vi "filter_frequency_imp_test_v10_p.vi"() -> ()   [LabVIEW 2014]
uses:
  <vilib>/rvi/Analysis/host/Butterworth/config/Butterworth Filter Order.ctl
  <vilib>/rvi/Analysis/host/Butterworth/config/Butterworth Filter Type.ctl
  <vilib>/FPGAPlugInAG/cRIO-9039/niLvFpga_Open_cRIO-9039.vi
  <vilib>/rvi/interface/common/dynamic/niFpgaDynamicAddResources.vi
  <vilib>/rvi/Analysis/host/Butterworth/config/BwScaledCoefficients.vi
  <vilib>/Utility/error.llb/Error Cluster From Error Code.vi
  <vilib>/rvi/errors/niLvFpgaAdjustHostInterfaceError.vi
  <vilib>/FPGAPlugInAG/Dynamic/niLvFpga_Close_Dynamic.vi
  <vilib>/rvi/interface/nirviOpenFPGA/nirviOpenFPGA.xnode
  FPGA Bitfiles/test0304_FPGATarget_imptestv10p1_N8vwftCNm6Q.lvbitx
  FPGA VIs/imp_test_v10_p1.vi
  <vilib>/rvi/Analysis/host/Butterworth/XNode/ButterworthCoefficients.xnode
  <vilib>/rvi/interface/nirviReadWriteControl/nirviReadWriteControl.xnode
  <vilib>/rvi/interface/nirviCloseFPGA/nirviCloseFPGA.xnode
  <vilib>/rvi/Analysis/host/Public/NI_FpgaMspHost.lvlib
  NiFpgaLv.dll
  <vilib>/rvi/interface/Simulation/niFpgaSimulationCallBeginRW.vi
panel:
  in  "sr_omega_p_Mavg (S/s)":dbl=50000.0
  in  "fcu_omega_p_Mavg (Hz)":dbl=1000.0
  in  "Filter set":bool
  in  "sr_Strain(Avg.8)_p (S/s)":dbl=50000.0
  in  "fcu_Strain(Avg.8)_p (Hz)":dbl=1000.0
  in  "sr_Dp_dd (S/s)":dbl=50000.0
  in  "fcu_Dp_dd (Hz)":dbl=1000.0
  in  "sr_dFp_PIS (S/s)":dbl=50000.0
  in  "fcu_dFp_PID (Hz)":dbl=1000.0
  in  "sr_Strain(Avg.8)_y (S/s)":dbl=50000.0
  in  "fcu_Strain(Avg.8)_y (Hz)":dbl=1000.0
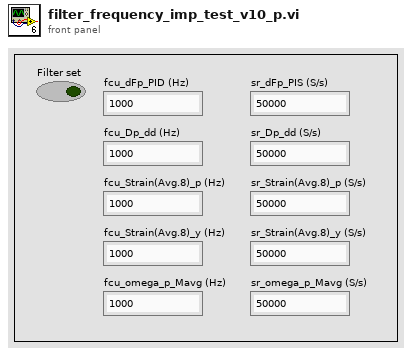
[diagram p1: front panel]
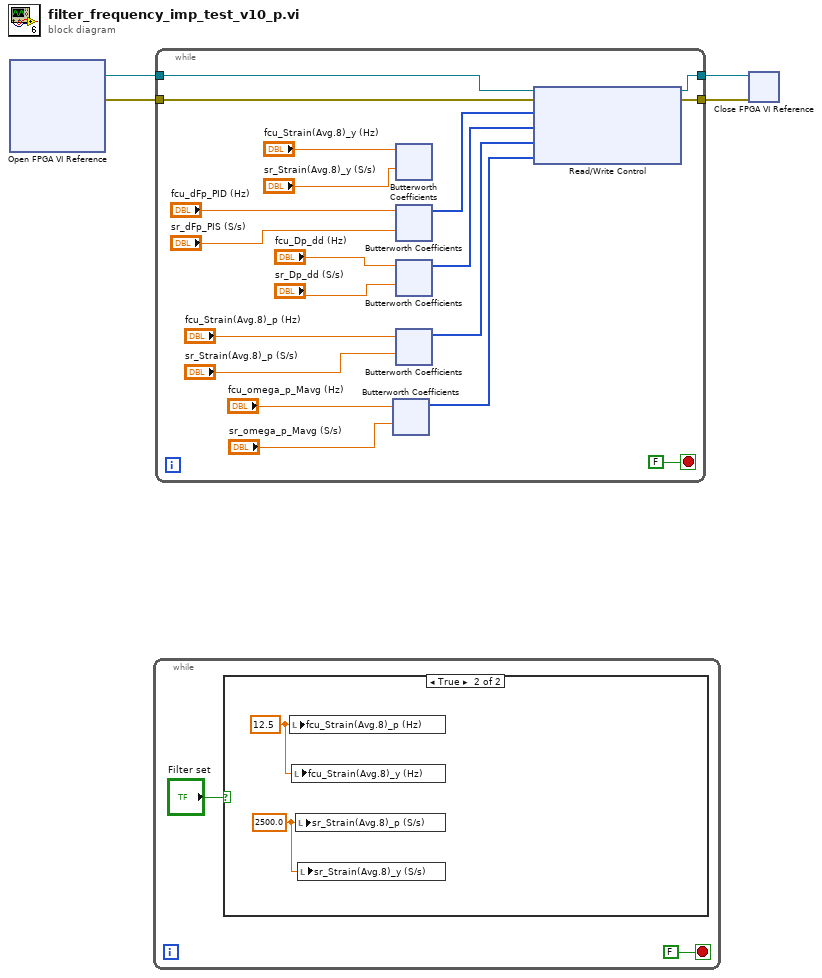
[diagram p0: block diagram]
diagram:
  n1 = xnode "Open FPGA VI Reference"() -> ("FPGA VI Reference Out"=w4:refnum<k20>, "error out"=w3:errorcluster)  [unwired: 2 in]
  n2 = while {
    stop <- FALSE stop-if-true
    n3 = case shown="True" "Filter set" {
      frame False {
      }
      frame True {
        w7 = 2500.0 ("sr_Strain(Avg.8)_p (S/s)")
        w8 = 12.5 ("fcu_Strain(Avg.8)_p (Hz)")
        n4 = local write "fcu_Strain(Avg.8)_p (Hz)"(w8) -> ()
        n5 = local write "fcu_Strain(Avg.8)_y (Hz)"(w8) -> ()
        n6 = local write "sr_Strain(Avg.8)_p (S/s)"(w7) -> ()
        n7 = local write "sr_Strain(Avg.8)_y (S/s)"(w7) -> ()
      }
    }
  }
  n8 = while {
    tunnel: w4 -> [w22]
    tunnel: w3 -> [w27]
    tunnel: [w26] -> w2
    tunnel: [w25] -> w1
    stop <- FALSE stop-if-true
    n9 = xnode "Butterworth Coefficients"("cutoff frequency (Hz)"="fcu_omega_p_Mavg (Hz)", "sample rate (S/s)"="sr_omega_p_Mavg (S/s)") -> ("scaled coefficients"=w12:i32[])  [unwired: 1 in, 1 out]
    n10 = xnode "Butterworth Coefficients"("cutoff frequency (Hz)"="fcu_Strain(Avg.8)_y (Hz)", "sample rate (S/s)"="sr_Strain(Avg.8)_y (S/s)") -> ()  [unwired: 1 in, 2 out]
    n11 = xnode "Butterworth Coefficients"("cutoff frequency (Hz)"="fcu_dFp_PID (Hz)", "sample rate (S/s)"="sr_dFp_PIS (S/s)") -> ("scaled coefficients"=w21:i32[])  [unwired: 1 in, 1 out]
    n12 = xnode "Butterworth Coefficients"("cutoff frequency (Hz)"="fcu_Dp_dd (Hz)", "sample rate (S/s)"="sr_Dp_dd (S/s)") -> ("scaled coefficients"=w20:i32[])  [unwired: 1 in, 1 out]
    n13 = xnode "Butterworth Coefficients"("cutoff frequency (Hz)"="fcu_Strain(Avg.8)_p (Hz)", "sample rate (S/s)"="sr_Strain(Avg.8)_p (S/s)") -> ("scaled coefficients"=w13:i32[])  [unwired: 1 in, 1 out]
    n14 = xnode "Read/Write Control"("FPGA VI Reference In"=w22, "error in"=w27, "dFp_PID coeff."=w21, "Dp_dd coeff."=w20, "Strain_p Avg.8 coeff."=w13, "omega_P(Mavg) coeff."=w12) -> ("FPGA VI Reference Out"=w26:refnum<k20>, "error out"=w25:errorcluster)
  }
  n15 = xnode "Close FPGA VI Reference"("FPGA VI Reference In"=w2, "error in"=w1) -> ()  [unwired: 1 out]
